vi "Check SDI Valid.vi"(10 "label settings for RT":T1 {"Label Timestamp Channel Data Reference" format="%.0x"; "Word Initial Raw Value" format="%032.0f"; "Label Disable/Trigger Channel Reference" format="%.0x"; "parameter driver data"."Tx parameter refs" format="%.0x"; "SDI" format="%02b"; "label" format="%.0o"}, 11 "data word in":u32) -> (2 "sdi valid?":bool, 3 "data word out":u32)   [LabVIEW 2020, in "AIM ARINC 429 Engine.lvlib" / "Implementation.lvlib" / "Rx Execution Unit.lvclass"]
uses:
  Rx Execution Unit.lvclass
  Shared/RT Label Settings.ctl
  Shared/Label.ctl
  Shared/RT Parameters.ctl
  Shared/Parameter Definition.ctl
  <vilib>/NI/NI VeriStand Encoding and Decoding/Encoding.ctl
  <vilib>/NI VeriStand/Custom Device API/Custom Device Item Ref.ctl
  Shared/Transfer Type.ctl
  <vilib>/NI VeriStand/Custom Device API/Data Reference.ctl
  <vilib>/NI VeriStand/Custom Device API/Custom Device API.lvlib
  <vilib>/NI/NI VeriStand Encoding and Decoding/Encoding and Decoding.lvlib
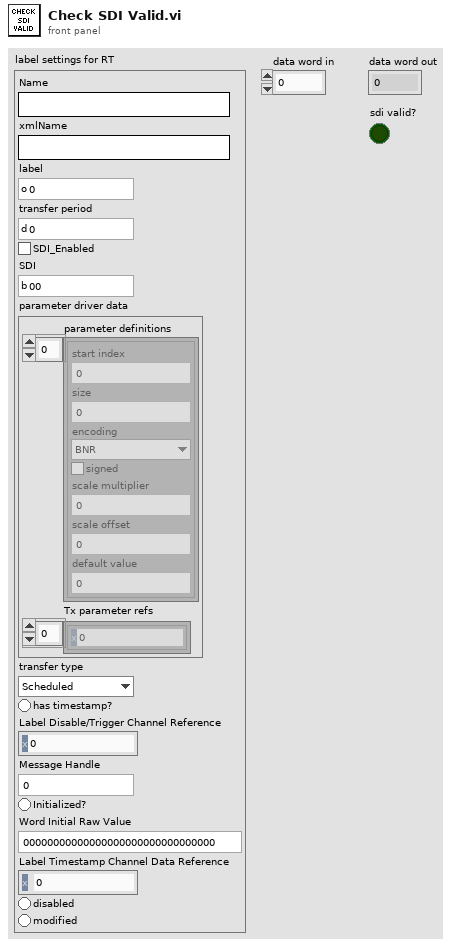
[diagram p1: front panel]
types:
  T1 = typedef "RT Label Settings.ctl" = cluster{"Name":string, "xmlName":string, "label":T2, "transfer period":u32, "SDI_Enabled":bool, "SDI":u8, "parameter driver data":T3, "transfer type":T7, "has timestamp?":bool, "Label Disable/Trigger Channel Reference":T6, "Message Handle":u64, "Initialized?":bool, "Word Initial Raw Value":u32, "Label Timestamp Channel Data Reference":T8, "disabled":bool, "modified":bool}
  T2 = typedef "Label.ctl" = u8
  T3 = typedef "RT Parameters.ctl" = cluster{"parameter definitions":T4[], "Tx parameter refs":T6[]}
  T4 = typedef "Parameter Definition.ctl" = cluster{"start index":i32, "size":i32, "encoding":T5, "signed":bool, "scale multiplier":dbl, "scale offset":dbl, "default value":dbl}
  T5 = typedef "Encoding and Decoding.lvlib/Encoding.ctl" = enum16{"BNR", "BCD", "Discrete"}
  T6 = typedef "Custom Device API.lvlib/Custom Device Item Ref.ctl" = u64
  T7 = typedef "Transfer Type.ctl" = enum16{"Scheduled", "Acyclic", "Block", "Strobe"}
  T8 = typedef "Custom Device API.lvlib/Data Reference.ctl" = i32
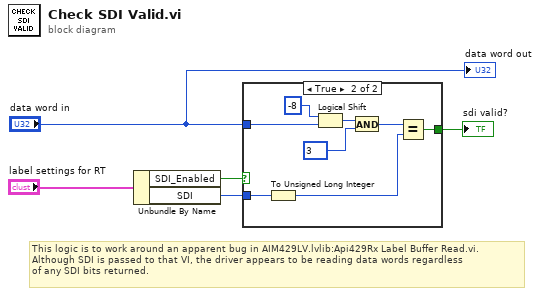
[diagram p0: block diagram]
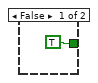
[diagram p2: hidden frame]
diagram:
  # "This logic is to work around an apparent bug in AIM429LV.lvlib:Api429Rx Label Buffer Read.vi.\nAlthough SDI is passed to that VI, the driver appears to be reading data words regardless\nof any SDI bits returned."
  n1 = Unbundle By Name("label settings for RT") -> ("SDI_Enabled"=w2:bool, "SDI"=w4:u8)
  n2 = case shown="True" w2 {
    tunnel: "data word in" -> [_ w10]
    tunnel: w4 -> [_ w14]
    tunnel: [TRUE w11] -> w1
    frame False {
    }
    frame True {
      n3 = To Unsigned Long Integer(number=w14) -> (unsigned 32bit integer=w8:u32)
      n4 = Logical Shift(y=i16 -8, x=w10) -> (x << y=w9:u32)
      n5 = And(x=w9, y=u32 3) -> (x .and. y?=w12:u32)
      n6 = Equal?(x=w12, y=w8) -> (x = y?=w11:bool)
    }
  }
  "sdi valid?" <- w1
  "data word out" <- "data word in"
